vi "Load_Channel_Config.vi"(8 "Error in":errorcluster, 10 "configuration file path":path) -> (0 "error out":errorcluster, 11 "Channel_Information":T1(array[cluster]) {"Input Terminal Configuration" items=["default"=-1, "RSE"=10083, "NRSE"=10078, "Differential"=10106, "Pseudodifferential"=12529]})   [LabVIEW 2017]
uses:
  <vilib>/Utility/config.llb/NI_LVConfig.lvlib
  <vilib>/Utility/config.llb/Read Key (String).vi
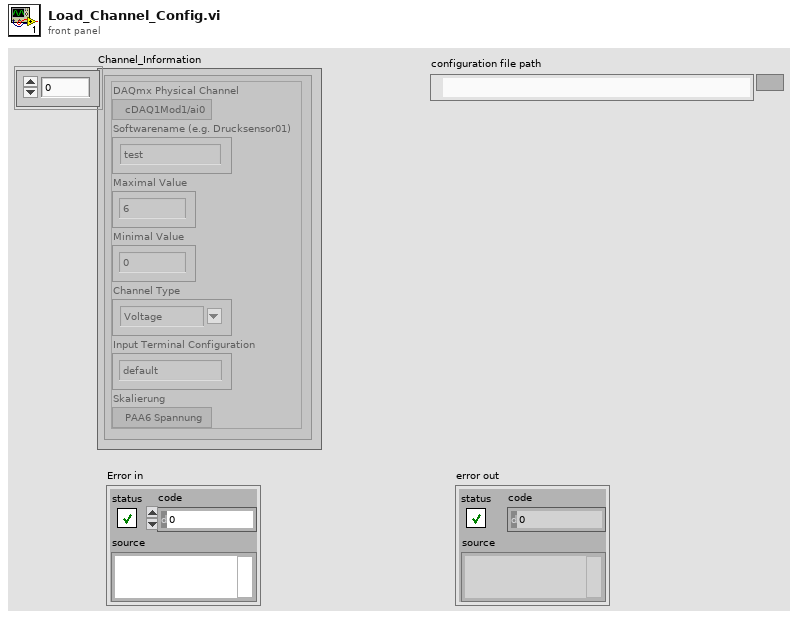
[diagram p1: front panel]
types:
  T1 = cluster{"DAQmx Physical Channel":tag, "Softwarename (e.g. Drucksensor01)":string, "Maximal Value":dbl, "Minimal Value":dbl, "Channel Type":string, "Input Terminal Configuration":i32, "Skalierung":tag}[]
  T2 = cluster{"DAQmx Physical Channel":tag, "Softwarename (e.g. Drucksensor01)":string, "Maximal Value":dbl, "Minimal Value":dbl, "Channel Type":string, "Input Terminal Configuration":i32, "Skalierung":tag}
  T3 = typedef "NI_LVConfig.lvlib/Config Data RefNum.ctl" = refnum<k1>
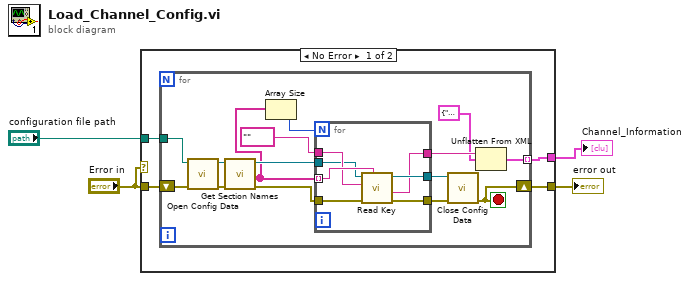
[diagram p0: block diagram]
diagram:
  n1 = case shown="No Error" "Error in" {
    tunnel: "Error in" -> [w8 w31]
    tunnel: "configuration file path" -> [w7 _]
    tunnel: [w6 w31] -> w3
    tunnel: [w5 _] -> w1
    frame No Error {
      n2 = for {
        tunnel: w7 -> [w22]
        shift-right: [w21] -> w6
        shift-left: w8 -> [w23]
        tunnel: [w12] -> w5 mode=indexing
        stop <- w21 stop-if-true
        n3 = call <vilib>:"Open Config Data.vi"("error in (no error)"=w23, "configuration file path"=w22) -> ("error out"=w16:errorcluster, "refnum"=w17:T3)  [unwired: 7 in, 1 out]
        n4 = call <vilib>:"Get Section Names.vi"("error in (no error)"=w16, "refnum"=w17) -> ("error out"=w18:errorcluster, "section names"=w10:string[], "refnum out"=w11:T3)  [unwired: 7 in]
        n5 = Array Size(array=w10) -> (size(s)=w9:i32)
        n6 = for {
          N: w9 -> [_]
          tunnel: [w30] -> w20
          tunnel: [w29] -> w19
          tunnel: w10 -> [w28] mode=indexing
          tunnel: w18 -> [w27]
          tunnel: [w26] -> w14
          tunnel: tag "" ("DAQmx Physical Channel") -> [w25]
          tunnel: w11 -> [w24]
          n7 = call-poly <vilib>:"Read Key.vi"("section"=w28, "error in (no error)"=w27, "key"=w25, "refnum"=w24) -> ("error out"=w30:errorcluster, "value"=w26:string, "refnum out"=w29:T3)  [unwired: 4 in, 1 out]
        }
        n8 = call <vilib>:"Close Config Data.vi"("error in (no error)"=w20, "refnum"=w19) -> ("error out"=w21:errorcluster)  [unwired: 8 in, 1 out]
        n9 = Unflatten From XML(xml string=w14, type=T2 {"DAQmx Physical Channel"="cDAQ1Mod1/ai0", "Softwarename (e.g. Drucksensor01)"="test", "Maximal Value"=6.0, "Minimal Value"=0.0, "Channel Type"="Voltage", "Input Terminal Configuration"=-1, "Skalierung"="PAA6 Spannung"} ("Channel_Information")) -> (value=w12:T2)  [unwired: 1 in, 1 out]
      }
    }
    frame Error {
    }
  }
  "Channel_Information" <- w1
  "error out" <- w3
